vi "Current Track INFO.vi"(0 "reference in":refnum<class "MediaPlayer.lvclass">, 11 "Error In":errorcluster) -> (4 "reference out":refnum<class "MediaPlayer.lvclass">, 6 "Name":string, 8 "Is playing?":bool, 15 "Error Out":errorcluster)   [LabVIEW 2024, in "MediaPlayer.lvclass"]
doc: "Get Current track info.\n- Name (str)\n- Duration (DBL)"
uses:
  MediaPlayer.lvclass
  MediaPlayer.lvclass/MediaPlayer.ctl
panel:
  # "Connector Pane"
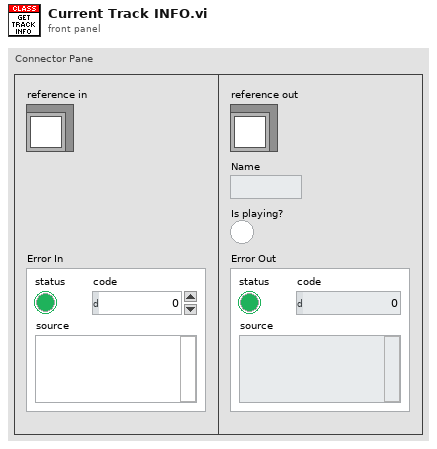
[diagram p1: front panel]
types:
  T1 = typedef "MediaPlayer.lvclass/ObjectAttributes.ctl" = cluster{"MediaPlayerData":T2}
  T2 = typedef "MediaPlayer.lvclass/MediaPlayer Data.ctl" = cluster{"Music List":path[], "Current Music Index":u16, "Song Handler":T3, "Device ID":u32}
  T3 = typedef "Sound Output Task ID.ctl" = u32
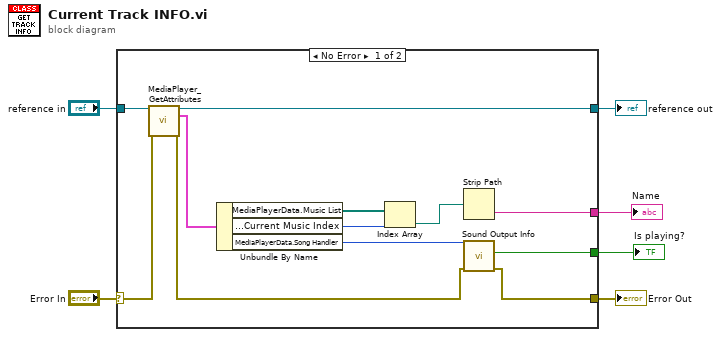
[diagram p0: block diagram]
diagram:
  n1 = case shown="No Error" "Error In" {
    selector: "Error In" -> [w18 w20]
    tunnel: [w7 w20] -> w5
    tunnel: [w15 w19] -> w3
    tunnel: "reference in" -> [w16 w19]
    tunnel: [w11 _] -> w2
    tunnel: [w9 _] -> w1
    frame No Error {
      n2 = call "MediaPlayer_GetAttributes.vi"("reference in"=w16, "Error In"=w18) -> ("reference out"=w15:refnum<class "MediaPlayer.lvclass">, "Data"=w17:T1, "Error Out"=w8:errorcluster)  [unwired: 10 in, 1 out]
      n3 = Unbundle By Name(w17) -> ("MediaPlayerData.Music List"=w13:path[], "MediaPlayerData.Current Music Index"=w14:u16, "MediaPlayerData.Song Handler"=w10:T3)
      n4 = Index Array(array=w13, index=w14) -> (element=w12:path)
      n5 = Strip Path(path=w12) -> (name=w11:string)  [unwired: 1 out]
      n6 = call <vilib>:"Sound Output Info.vi"("error in (no error)"=w8, "task ID"=w10) -> ("error out"=w7:errorcluster, "is playing?"=w9:bool)  [unwired: 6 in, 2 out]
    }
    frame Error {
    }
  }
  "Error Out" <- w5
  "reference out" <- w3
  "Name" <- w2
  "Is playing?" <- w1
